vi "Wait for Completion.vi"(8 "error in (no error)":errorcluster, 9 "Timeout":i32, 11 "Coverage Analyzer Process in":refnum<class "Coverage Analyzer Process.lvclass">) -> (0 "error out":errorcluster, 3 "Coverage Analyzer Process out":refnum<class "Coverage Analyzer Process.lvclass">)   [LabVIEW 2020, in "Coverage Analyzer.lvlib" / "Coverage Analyzer Process.lvclass"]
uses:
  Coverage Analyzer Process.lvclass
  Coverage Analyzer Result View/Coverage Analyzer View Data.ctl
  Coverage Analyzer Process.lvclass/Coverage Analyzer Process.ctl
  Coverage Analyzer Result View/Coverage Analyzer View.vi
  Coverage Analyzer Result View/Coverage Analyzer Result View.lvclass
  Coverage Analyzer/Coverage Analyzer.lvclass
panel:
  in  "Suite Result":bool
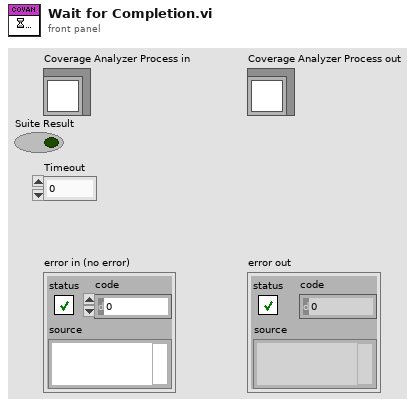
[diagram p1: front panel]
types:
  T1 = typedef "Coverage Analyzer.lvlib/Coverage Analyzer Result View.lvclass/Coverage Analyzer View Data.ctl" = cluster{"Code Coverage":map{path, dbl}}
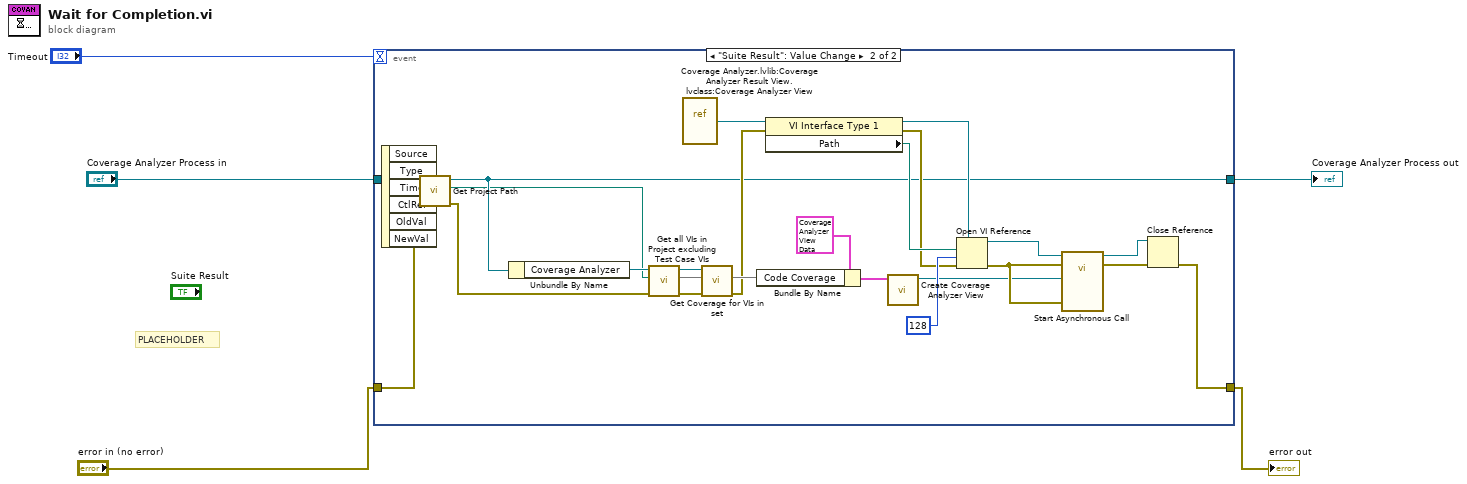
[diagram p0: block diagram]
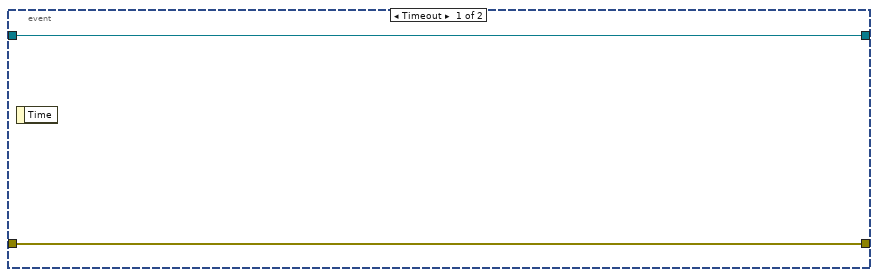
[diagram p2: hidden frame]
diagram:
  # "PLACEHOLDER"
  n1 = event shown="[1] \"Suite Result\": Value Change" {
    selector: _ -> [_ _]
    dyn-events: _ -> [_ _]
    timeout: "Timeout" -> [_ _]
    tunnel: "error in (no error)" -> [w7 w12]
    tunnel: [w7 w22] -> w3
    tunnel: "Coverage Analyzer Process in" -> [w6 w14]
    tunnel: [w6 w15] -> w1
    event Timeout {
      n2 = event-data() -> ()  [unwired: 1 in, 1 out]
    }
    event "Suite Result": Value Change {
      n3 = event-data() -> ()  [unwired: 1 in, 6 out]
      n4 = call "Get Project Path.vi"("error in (no error)"=w12, "Coverage Analyzer Process in"=w14) -> ("error out"=w13:errorcluster, "Path"=w9:path, "Coverage Analyzer Process out"=w15:refnum<class "Coverage Analyzer Process.lvclass">)  [unwired: 7 in]
      n5 = Unbundle By Name(w15) -> ("Coverage Analyzer"=w20:refnum<class "Coverage Analyzer.lvclass">)
      n6 = call "Get all VIs in Project excluding Test Case VIs.vi"("error in (no error)"=w13, "Path"=w9, "Coverage Analyzer in"=w20) -> ("error out"=w17:errorcluster, "VIs"=w8:set{path}, "Coverage Analyzer out"=w19:refnum<class "Coverage Analyzer.lvclass">)  [unwired: 6 in]
      n7 = vi-ref "Coverage Analyzer.lvlib:Coverage Analyzer Result View.lvclass:Coverage Analyzer View.vi"() -> (w24:refnum<vi>)
      n8 = call "Get Coverage for VIs in set.vi"("error in (no error)"=w17, "VIs"=w8, "Coverage Analyzer in"=w19) -> ("error out"=w16:errorcluster, "Code Coverage"=w18:map{path, dbl})  [unwired: 6 in, 1 out]
      n9 = Bundle By Name(cluster=T1 {"Code Coverage"={}} ("Data"), "Code Coverage"=w18) -> (w11:T1)
      n10 = property class="VI Interface Type 1"(reference=w24, error in=w16) -> (reference out=w28:refnum<vi>, error out=w26:errorcluster, "Path"=w27:path)
      n11 = call "Create Coverage Analyzer View.vi"("Coverage Analyzer Result View in"=w11) -> ("Coverage Analyzer Result View out"=w10:refnum<class "Coverage Analyzer Result View.lvclass">)  [unwired: 9 in, 1 out]
      n12 = Open VI Reference(type specifier VI Refnum (for type only)=w28, vi path=w27, options=128, error in (no error)=w26) -> (vi reference=w23:refnum<vi>, error out=w25:errorcluster)  [unwired: 2 in]
      n13 = call-by-ref "Start Asynchronous Call"(reference=w23, error in=w25, 8:"error in (no error)"=w25, "Coverage Analyzer Result View.lvclass"=w10) -> (reference out=w31:refnum<vi>, error out=w30:errorcluster)  [unwired: 9 in, 1 out]
      n14 = Close Reference(reference=w31, error in (no error)=w30) -> (error out=w22:errorcluster)
    }
  }
  "error out" <- w3
  "Coverage Analyzer Process out" <- w1
